vi "FPGAztrajectory.vi"(1 "z step size derived":u16, 2 "z amplitude":u16, 3 "z/intensity memory address":u32) -> (0 "Z trajectory":i16)   [LabVIEW 2010]
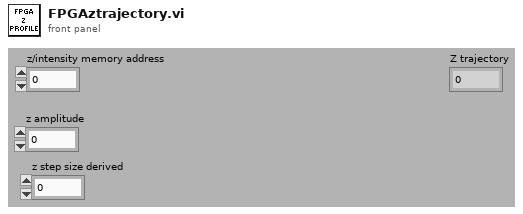
[diagram p1: front panel]
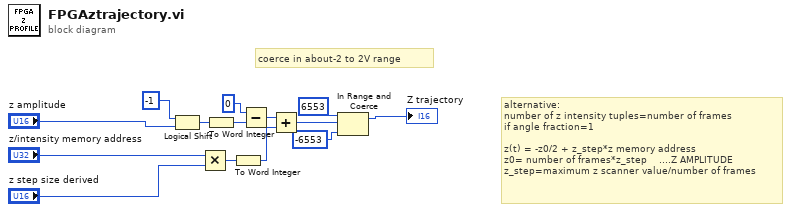
[diagram p0: block diagram]
diagram:
  # "alternative:\nnumber of z intensity tuples=number of frames\nif angle fraction=1\n\nz(t) = -z0/2 + z_step*z memory address\nz0= number of frames*z_step    ....Z AMPLITUDE\nz_step=maximum z scanner value/number of frames"
  # "coerce in about-2 to 2V range"
  n1 = Logical Shift(y=i16 -1 ("n"), x="z amplitude") -> (x << y=w13:u16)
  n2 = Multiply(x="z/intensity memory address", y="z step size derived") -> (x*y=w5:u32)
  n3 = To Word Integer(number=w13) -> (16bit integer=w6:i16)
  n4 = To Word Integer(number=w5) -> (16bit integer=w7:i16)
  n5 = Subtract(x=i16 0, y=w6) -> (x-y=w4:i16)
  n6 = Add(x=w4, y=w7) -> (x+y=w10:i16)
  n7 = In Range and Coerce(upper limit=i16 6553, x=w10, lower limit=i16 -6553) -> (coerced(x)=→"Z trajectory":i16)  [unwired: 1 out]
